vi "parts.vi"   [LabVIEW 2011]
uses:
  <vilib>/Quanser/Rapid Control Prototyping Toolkit/visualization/Visualization Set Variable.vi
  <vilib>/Quanser/Rapid Control Prototyping Toolkit/visualization/Visualization.lvclass
  <vilib>/Quanser/Rapid Control Prototyping Toolkit/visualization/Visualization Set Variable (SGL).vi
  <vilib>/Quanser/Rapid Control Prototyping Toolkit/visualization/Visualization Select Variable (2D SGL).vi
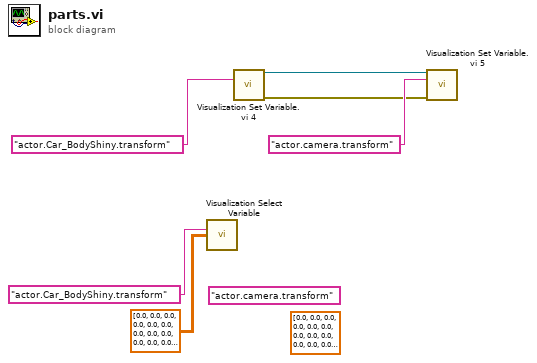
[diagram p0: block diagram]
diagram:
  w1 = sgl[][] [[0.0, 0.0, 0.0, 0.0], [0.0, 0.0, 0.0, 0.0], [0.0, 0.0, 0.0, 0.0], [0.0, 0.0, 0.0, 0.0]] ("initial value")
  w5 = "actor.camera.transform" ("variable name")
  n1 = call-poly <vilib>:"Visualization Select Variable.vi"("variable name"="actor.Car_BodyShiny.transform", "initial values"=sgl[][] [[0.0, 0.0, 0.0, 0.0], [0.0, 0.0, 0.0, 0.0], [0.0, 0.0, 0.0, 0.0], [0.0, 0.0, 0.0, 0.0]] ("initial value")) -> ("visualization out"=w3:refnum<class "Visualization.lvclass">, "error in (no error)"=w2:errorcluster, "error out"=w4:errorcluster)  [unwired: 11 in]
  n2 = call-poly "Visualization Set Variable.vi 4"("variable name"="actor.Car_BodyShiny.transform") -> ("visualization out"=w11:refnum<class "Visualization.lvclass">, "value"=w9:sgl, "error out"=w10:errorcluster)  [unwired: 12 in]
  n3 = call-poly "Visualization Set Variable.vi 5"("visualization in"=w11, "variable name"="actor.camera.transform", "error in (no error)"=w10) -> ("value"=w8:sgl)  [unwired: 10 in, 2 out]
